vi "Valid units Write.vi"(4 "error in (no error)":errorcluster, 5 "Value":T1[](array[typedef]), 6 "Container State":T3, 7 "Display State In":T2) -> (0 "error out":errorcluster, 3 "Display State Out":T2)   [LabVIEW 2015, in "Level (G3).xctl"]
uses:
  Level (G3).xctl
  <vilib>/_xctls/Container State.ctl
  State.ctl
  Utility VIs/Controls/KRing/KRing.xctl
  Utility VIs/Controls/KNumeric (DBL)/KNumeric (DBL).xctl
  Level Units (G3).ctl
  <vilib>/_xctls/XControlSupport.lvlib
panel:
  in  "Units":T1
  # "Replace the Value Control below with a Control of desired type.\nDo not remove this Control or the others from the connector pane.\nDo not change the connector pane pattern.\nThe Value control should always be the third terminal from top on the input side in the connector pane."
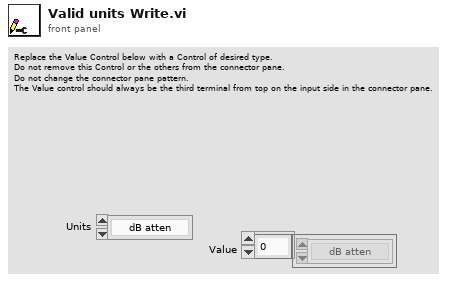
[diagram p1: front panel]
types:
  T1 = typedef "Level (G3).xctl/Level Units (G3).ctl" = enum16{"dB atten", "dB SPL", "dB re 1 Vrms", "dB V/Hz½", "dB SL", "mW", "Volts"}
  T2 = typedef "Level (G3).xctl/State.ctl" = cluster{"LMax Event":refnum<user-event>, "enable menu":bool, "Units":string[], "Valid":bool[], "multi":bool, "ctl":cluster{"Units":refnum<vi>, "Level":refnum<vi>}}
  T3 = typedef "XControlSupport.lvlib/Container State.ctl" = cluster{"Indicator?":bool, "Run Mode?":bool, " Refnum":refnum<vi>}
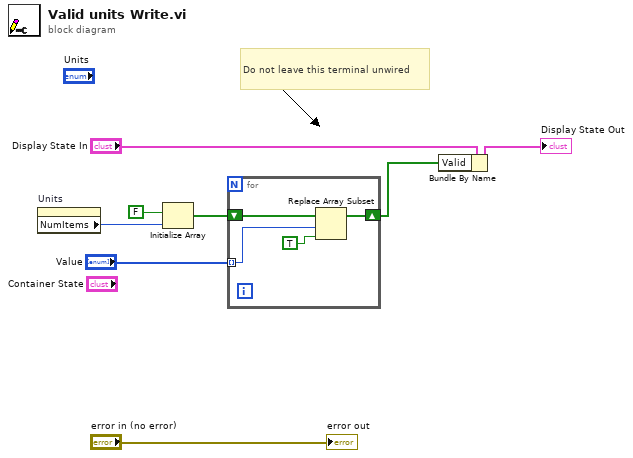
[diagram p0: block diagram]
diagram:
  # "Do not leave this terminal unwired"
  n1 = property on="Units" class="Enum (strict)"() -> ("NumItems"=w6:u32)  [unwired: 2 in, 2 out]
  n2 = Initialize Array(FALSE, w6) -> (w3:bool[])
  n3 = for {
    tunnel: "Value" -> [w10] mode=indexing
    shift-right: [w11] -> w1
    shift-left: w3 -> [w12]
    n4 = Replace Array Subset(array=w12, new element=TRUE, index=w10) -> (w11:bool[])
  }
  n5 = Bundle By Name(cluster="Display State In", "Valid"=w1) -> (→"Display State Out":T2)
  "error out" <- "error in (no error)"
